vi "Procedure - Send Data.vi"(0 "Procedure Step":T1, 1 "Wait Ticks Remaining":u32, 2 "CMD Length [1-40]":u8, 5 "SRL Wait Ticks":u32, 7 "Write Bit Index [0-18]":u8, 9 "SRL Cycle Mode":bool, 11 "error in (no error)":errorcluster, 12 "SRL Cycle CMD":u64, 13 "Socket Mask":u32) -> (3 "Wait Ticks Remaining Out":u32, 4 "Procedure Step Out":T1, 8 "Write Bit Index [0-18] Out":u8, 10 "Finished":bool, 15 "error out":errorcluster)   [LabVIEW 2017, in "FPGA-SRL.lvlib"]
uses:
  FPGA-SRL.lvlib
  Type Defs/WSVCAP SHL Procedure Step Enum.ctl
  Type Defs/Write Line Enum.ctl
  Type Defs/WSVCAP SHL FIFO Operation Enum.ctl
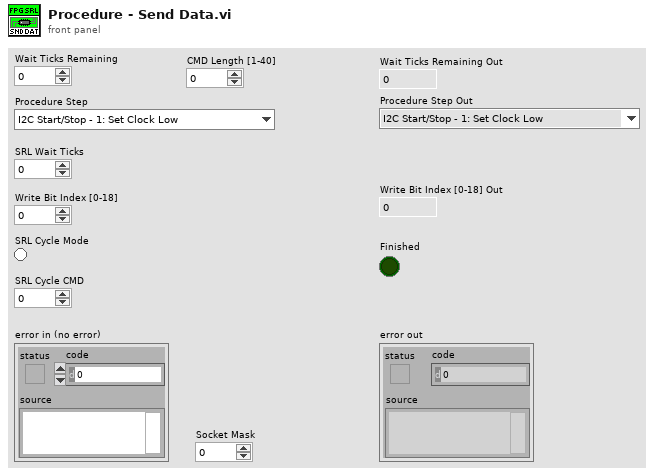
[diagram p1: front panel]
types:
  T1 = typedef "WSVCAP SHL Procedure Step Enum.ctl" = enum16{"I2C Start/Stop - 1: Set Clock Low", "I2C Start/Stop - 2: Wait", "I2C Start/Stop - 3: Set Data I", "I2C Start/Stop - 4: Wait", "I2C Start/Stop - 5: Set Clock High", "I2C Start/Stop - 6: Wait", "I2C Start/Stop - 7: Set Data II", "I2C Start/Stop - 8: Wait", "I2C Start/Stop - 9: Set Clock Low", "I2C Start/Stop - 10: Wait", "I2C Read ACK - 1: Set Clock High", "I2C Read ACK - 2: Wait", "I2C Read ACK - 3: Read ACK Bit", "I2C Read ACK - 4: Wait", "I2C Read ACK - 5: Set Clock Low", "I2C Read ACK - 6: Wait", "I2C Write ACK - 1: Write ACK Bit", "I2C Write ACK - 2: Wait", "I2C Write ACK - 3: Set Clock High", "I2C Write ACK - 4: Wait", "I2C Write ACK - 5: Set Clock Low", "I2C Write ACK - 6: Wait", "I2C Write ACK - 7: Set Data Low", "I2C Send Add - 1: Reset Bits Remaining", "I2C Send Add - 2: Set Data Bit", "I2C Send Add - 3: Wait", "I2C Send Add - 4: Set Clock High", "I2C Send Add - 5: Wait", "I2C Send Add - 6: Set Clock Low", "I2C Send Add - 7: Wait", "I2C Send Add - 8: Check Bits Remaining", "I2C Send Data - 1: Reset Bits Remaining", "I2C Send Data - 2: Load Write Bit from FIFO", "I2C Send Data - 3: Set Data Bit", "I2C Send Data - 4: Wait", "I2C Send Data - 5: Set Clock High", "I2C Send Data - 6: Wait", "I2C Send Data - 7: Set Clock Low", "I2C Send Data - 8: Wait", "I2C Send Data - 9: Check Bits Remaining", "I2C Receive Data - 1: Reset Bits Remaining", "I2C Receive Data - 2: Wait", "I2C Receive Data - 3: Set Clock High", "I2C Receive Data - 4: Wait", "I2C Receive Data - 5: Read Data Bit", "I2C Receive Data - 6: Wait", "I2C Receive Data - 7: Set Clock Low", "I2C Receive Data - 8: Wait", "I2C Receive Data - 9: Check Bits Remaining", "RFFE Send SSC - 1:Set Low", "RFFE Send SSC - 2:Wait", "RFFE Send SSC - 3:Set SDA High", "RFFE Send SSC - 4:Wait", "RFFE Send SSC - 5:Set SDA Low", "RFFE Send SSC - 6:Wait", "RFFE Send Data - 1:Set SCL High", "RFFE Send Data - 2:Wait", "RFFE Send Data - 3:Set SCL Low", "RFFE Send Data - 4:Wait", "RFFE Send Data - 5:Set SCL High (P)", "RFFE Send Data - 6:Wait", "RFFE Send Data - 7:Set SCL Low (P)", "RFFE Send Data - 8:Wait", "RFFE Send Data - 9:Set SCL High (BP)", "RFFE Send Data - 10:Wait", "RFFE Send Data - 11:Set SCL Low (BP)", "RFFE Send Data - 12:Wait", "RFFE Receive Data - 1:Set SCL High", "RFFE Receive Data - 2:Wait", "RFFE Receive Data - 3:Set SCL Low", "RFFE Receive Data - 4:Wait", "RFFE Receive Data - 5:Set SCL High (BP)", "RFFE Receive Data - 6:Wait", "RFFE Receive Data - 7:Set SCL Low (BP)", "RFFE Receive Data - 8:Wait", "RFFE Wait CMD Delay - 1:Wait", "RFFE Clear Lines - 1:Clear", "SRL Write Data - 1:Set SYNC High", "SRL Write Data - 2:Wait SYNC Delay", "SRL Write Data - 3:Set SYNC Low", "SRL Write Data - 4:Set SCLK High", "SRL Write Data - 5:Wait", "SRL Write Data - 6:Set SCLK Low", "SRL Write Data - 7:Wait", "SRL Write Data - 8:Set SYNC High", "SRL Wait CMD Delay - 1:Wait", "SRL Clear Lines - 1:Clear"}
  T2 = typedef "FPGA-SRL.lvlib/Write Line Enum.ctl" = enum16{"DIN", "SYNC", "SCLK"}
  T3 = typedef "WSVCAP SHL FIFO Operation Enum.ctl" = enum16{"Create FIFO/Memory", "Get Write FIFO Status", "Get Read FIFO Status", "Put Element in Write", "Put Element in Read", "Get Element from Write", "Get Element from Read"}
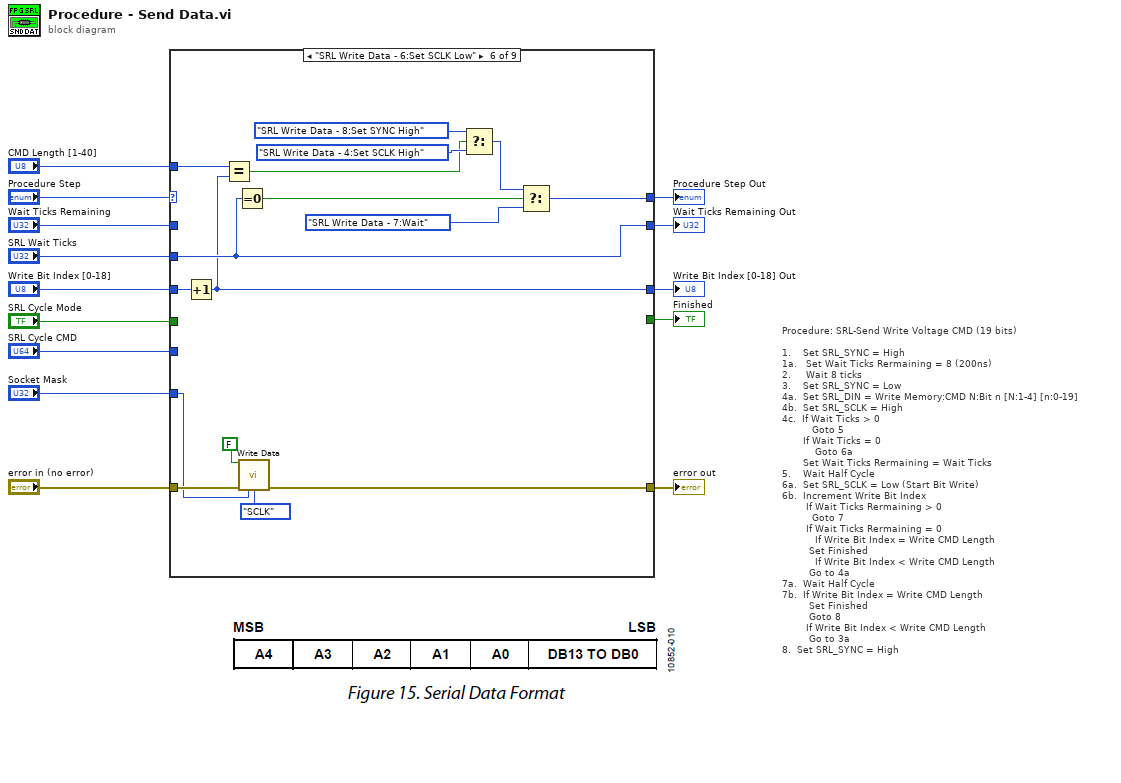
[diagram p0: block diagram]
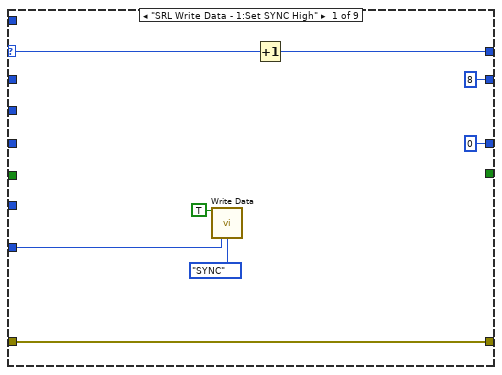
[diagram p2: hidden frame]
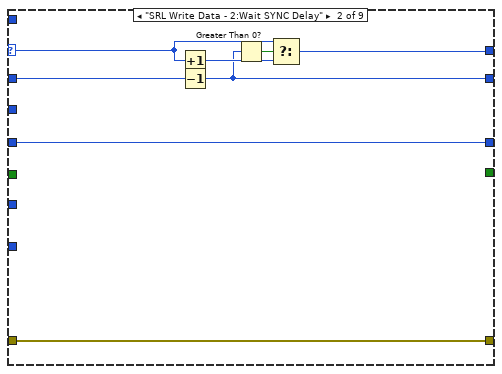
[diagram p3: hidden frame]
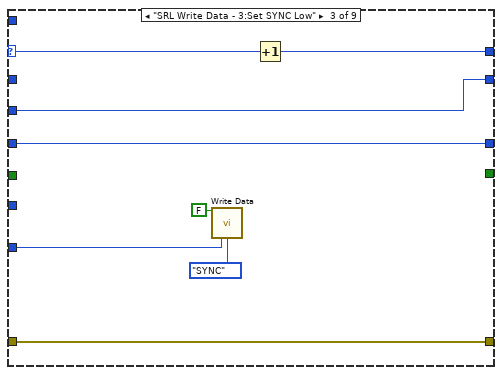
[diagram p4: hidden frame]
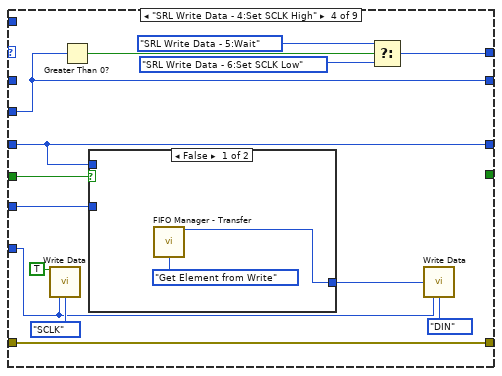
[diagram p5: hidden frame]
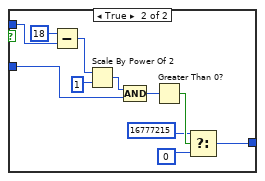
[diagram p6: hidden frame]
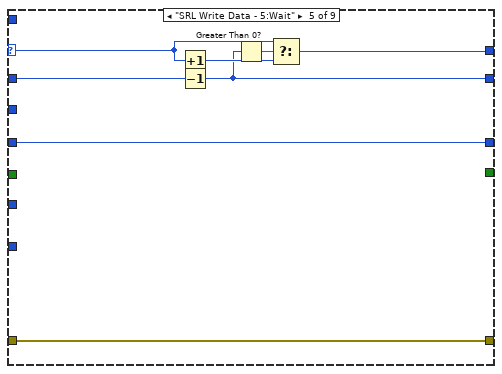
[diagram p7: hidden frame]
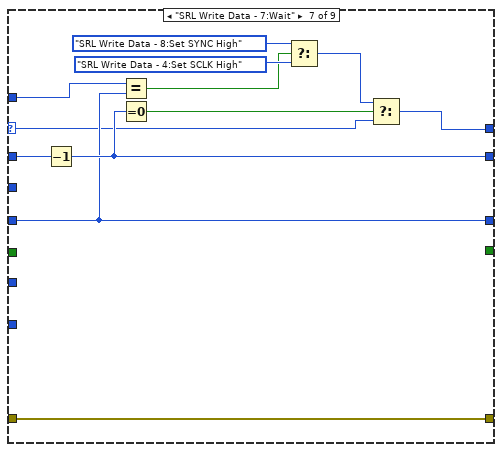
[diagram p8: hidden frame]
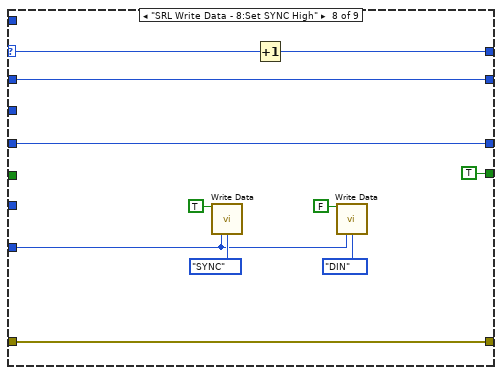
[diagram p9: hidden frame]
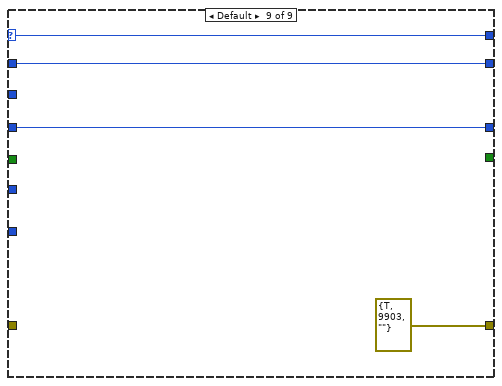
[diagram p10: hidden frame]
diagram:
  # "Procedure: SRL-Send Write Voltage CMD (19 bits)\n\n1.    Set SRL_SYNC = High\n1a.   Set Wait Ticks Rermaining = 8 (200ns)\n2.     Wait 8 ticks\n3.    Set SRL_SYNC = Low\n4a.  Set SRL_DIN = Write Memory:CMD N:Bit n [N:1-4] [n:0-19]\n4b.  Set SRL_SCLK = High\n4c.  If Wait Ticks > 0\n          Goto 5\n       If Wait Ticks = 0 \n           Goto 6a\n       Set Wait Ticks Rermaining = Wait Ticks\n5.    Wait Half Cycle\n6a.  Set SRL_SCLK = Low (Start Bit Write)\n6b.  Increment Write Bit Index\n        If Wait Ticks Rermaining > 0\n          Goto 7\n        If Wait Ticks Rermaining = 0 \n           If Write Bit Index = Write CMD Length\n         Set Finished\n           If Write Bit Index < Write CMD Length\n         Go to 4a\n7a.  Wait Half Cycle\n7b.  If Write Bit Index = Write CMD Length\n         Set Finished\n         Goto 8\n        If Write Bit Index < Write CMD Length\n         Go to 3a\n8.  Set SRL_SYNC = High"
  n1 = case shown="\"SRL Write Data - 6:Set SCLK Low\"" "Procedure Step" {
    selector: "Procedure Step" -> [w20 w28 w36 _ w71 _ w92 w110 w115]
    tunnel: [w17 w30 w33 w46 w73 w86 w101 w106 errorcluster {"status"=TRUE, "code"=9903, "source"=""} ("error IO")] -> w13
    tunnel: "error in (no error)" -> [w17 w30 w33 w46 w73 w87 w101 w106 _]
    tunnel: "Wait Ticks Remaining" -> [_ w26 _ _ w69 _ w100 w108 w114]
    tunnel: "SRL Wait Ticks" -> [_ _ w32 w40 _ w81 _ _ _]
    tunnel: [_ _ _ _ _ _ _ TRUE _] -> w12
    tunnel: "Write Bit Index [0-18]" -> [_ w23 w31 w39 w66 w83 w93 w107 w113]
    tunnel: "Socket Mask" -> [w18 _ w34 w48 _ w85 _ w102 _]
    tunnel: "SRL Cycle Mode" -> [_ _ _ w45 _ _ _ _ _]
    tunnel: "SRL Cycle CMD" -> [_ _ _ w44 _ _ _ _ _]
    tunnel: "CMD Length [1-40]" -> [_ _ _ _ _ w84 w99 _ _]
    tunnel: [w19 w25 w35 w41 w68 w82 w97 w109 w115] -> w4
    tunnel: [u32 8 ("Wait Ticks Remaining") w24 w32 w40 w67 w81 w96 w108 w114] -> w3
    tunnel: [u8 0 ("Write Bit Index [0-19]") w23 w31 w39 w66 w74 w93 w107 w113] -> w2
    frame "SRL Write Data - 1:Set SYNC High" {
      n2 = call "Write Data.vi"("Bit In (SCLK & SYNC)"=TRUE ("Bit In"), "Socket Mask"=w18, "Line"=Write_Line_Enum."SYNC") -> ()  [unwired: 12 in, 1 out]
      n3 = Increment(x=w20) -> (x+1=w19:T1)
    }
    frame "SRL Write Data - 2:Wait SYNC Delay" {
      n4 = Increment(x=w28) -> (x+1=w27:T1)
      n5 = Decrement(x=w26) -> (x-1=w24:u32)
      n6 = Greater Than 0?(x=w24) -> (x > 0?=w29:bool)
      n7 = Select(t=w28, s=w29, f=w27) -> (s? t:f=w25:T1)
    }
    frame "SRL Write Data - 3:Set SYNC Low" {
      n8 = call "Write Data.vi"("Bit In (SCLK & SYNC)"=FALSE ("Bit In"), "Socket Mask"=w34, "Line"=Write_Line_Enum."SYNC") -> ()  [unwired: 12 in, 1 out]
      n9 = Increment(x=w36) -> (x+1=w35:T1)
    }
    frame "SRL Write Data - 4:Set SCLK High" {
      n10 = call "Write Data.vi"("Bit In (SCLK & SYNC)"=TRUE ("Bit In"), "Socket Mask"=w48, "Line"=Write_Line_Enum."SCLK") -> ()  [unwired: 12 in, 1 out]
      n11 = Greater Than 0?(x=w40) -> (x > 0?=w49:bool)
      n12 = case shown="False" w45 {
        tunnel: [w53 w59] -> w47
        tunnel: w44 -> [_ w58]
        tunnel: w39 -> [_ w56]
        frame False {
          n13 = call "FIFO Manager - Transfer.vi"("Operation"=WSVCAP_SHL_FIFO_Operation_Enum."Get Element from Write") -> ("Data Out"=w53:u32)  [unwired: 12 in, 2 out]
        }
        frame True {
          n14 = Subtract(x=u8 18 ("y"), y=w56) -> (x-y=w55:u8)
          n15 = Scale By Power Of 2(n=w55, x=u64 1 ("Data Out")) -> (x*2^n=w64:u64)
          n16 = Compound Arithmetic op=AND(w64, w58) -> (w63:u64)
          n17 = Greater Than 0?(x=w63) -> (x > 0?=w62:bool)
          n18 = Select(t=u32 16777215 ("Data Out"), s=w62, f=u32 0 ("Data Out")) -> (s? t:f=w59:u32)
        }
      }
      n19 = Select(t=WSVCAP_SHL_Procedure_Step_Enum."SRL Write Data - 5:Wait" ("Procedure Step"), s=w49, f=WSVCAP_SHL_Procedure_Step_Enum."SRL Write Data - 6:Set SCLK Low" ("Procedure Step")) -> (s? t:f=w41:T1)
      n20 = call "Write Data.vi"("Word In (DIN)"=w47, "Socket Mask"=w48, "Line"=Write_Line_Enum."DIN") -> ()  [unwired: 12 in, 1 out]
    }
    frame "SRL Write Data - 5:Wait" {
      n21 = Increment(x=w71) -> (x+1=w70:T1)
      n22 = Decrement(x=w69) -> (x-1=w67:u32)
      n23 = Greater Than 0?(x=w67) -> (x > 0?=w72:bool)
      n24 = Select(t=w71, s=w72, f=w70) -> (s? t:f=w68:T1)
    }
    frame "SRL Write Data - 6:Set SCLK Low" {
      n25 = Increment(x=w83) -> (x+1=w74:u8)
      n26 = Equal?(x=w84, y=w74) -> (x = y?=w77:bool)
      n27 = Equal To 0?(x=w81) -> (x = 0?=w78:bool)
      n28 = call "Write Data.vi"("Bit In (SCLK & SYNC)"=FALSE ("Bit In"), "error in (no error)"=w87, "Socket Mask"=w85, "Line"=Write_Line_Enum."SCLK") -> ("error out"=w86:errorcluster)  [unwired: 11 in]
      n29 = Select(t=WSVCAP_SHL_Procedure_Step_Enum."SRL Write Data - 8:Set SYNC High" ("Procedure Step"), s=w77, f=WSVCAP_SHL_Procedure_Step_Enum."SRL Write Data - 4:Set SCLK High" ("Procedure Step")) -> (s? t:f=w76:T1)
      n30 = Select(t=w76, s=w78, f=WSVCAP_SHL_Procedure_Step_Enum."SRL Write Data - 7:Wait" ("Procedure Step")) -> (s? t:f=w82:T1)
    }
    frame "SRL Write Data - 7:Wait" {
      n31 = Decrement(x=w100) -> (x-1=w96:u32)
      n32 = Equal?(x=w99, y=w93) -> (x = y?=w91:bool)
      n33 = Equal To 0?(x=w96) -> (x = 0?=w98:bool)
      n34 = Select(t=WSVCAP_SHL_Procedure_Step_Enum."SRL Write Data - 8:Set SYNC High" ("Procedure Step"), s=w91, f=WSVCAP_SHL_Procedure_Step_Enum."SRL Write Data - 4:Set SCLK High" ("Procedure Step")) -> (s? t:f=w90:T1)
      n35 = Select(t=w90, s=w98, f=w92) -> (s? t:f=w97:T1)
    }
    frame "SRL Write Data - 8:Set SYNC High" {
      n36 = call "Write Data.vi"("Bit In (SCLK & SYNC)"=TRUE ("Bit In"), "Socket Mask"=w102, "Line"=Write_Line_Enum."SYNC") -> ()  [unwired: 12 in, 1 out]
      n37 = Increment(x=w110) -> (x+1=w109:T1)
      n38 = call "Write Data.vi"("Bit In (SCLK & SYNC)"=FALSE ("Bit In"), "Socket Mask"=w102, "Line"=Write_Line_Enum."DIN") -> ()  [unwired: 12 in, 1 out]
    }
    frame Default {
    }
  }
  "error out" <- w13
  "Finished" <- w12
  "Procedure Step Out" <- w4
  "Wait Ticks Remaining Out" <- w3
  "Write Bit Index [0-18] Out" <- w2
